vi "Expand.vi"(8 "error in (no error)":errorcluster, 10 "IB_Tree.lvclass":refnum<class "IB_Tree.lvclass">, 11 "IB_TreeProjFolder in":refnum<class "IB_Tree_Item_Proj_Folder.lvclass">) -> (0 "error out":errorcluster, 2 "first expansion?":bool, 3 "IB_TreeProjFolder out":refnum<class "IB_Tree_Item_Proj_Folder.lvclass">)   [LabVIEW 2020, in "IB_Tree_Item_Proj_Folder.lvclass"]
uses:
  <vilib>/AppBuilder/IB_Classes/Tree_Item_Proj_Folder/IB_Tree_Item_Proj_Folder.lvclass
  <vilib>/AppBuilder/IB_Classes/Tree_Item_Proj_Folder/IB_Tree_Item_Proj_Folder.lvclass/IB_Tree_Item_Proj_Folder.ctl
  <vilib>/AppBuilder/IB_Classes/Tree_Item/IB_Tree_Item.lvclass
  <vilib>/AppBuilder/IB_Classes/Tree_Item_Proj/IB_Tree_Item_Proj.lvclass
  <vilib>/AppBuilder/IB_Classes/Tree/IB_Tree.lvclass
  <vilib>/AppBuilder/IB_Classes/Tree_Item_Proj_Container/IB_Tree_Item_Proj_Container.lvclass
  e:/builds/penguin/labview/branches/2020/dev/dist/vi.lib/AppBuilder/IB_Classes/Tree_Item_Proj_Container/IB_Tree_Item_Proj_Container.lvclass
  e:/builds/penguin/labview/branches/2020/dev/dist/vi.lib/AppBuilder/IB_Classes/Tree_Item_Proj/IB_Tree_Item_Proj.lvclass
  e:/builds/penguin/labview/branches/2020/dev/dist/vi.lib/AppBuilder/IB_Classes/Tree_Item/IB_Tree_Item.lvclass
  e:/builds/penguin/labview/branches/2020/dev/dist/vi.lib/AppBuilder/IB_Classes/Tree_Item_Proj_Folder/IB_Tree_Item_Proj_Folder.lvclass
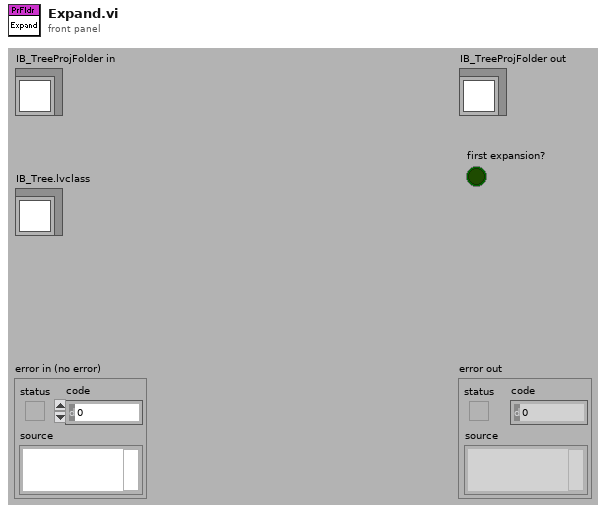
[diagram p1: front panel]
types:
  T1 = typedef "IB_Tree_Item.ctl" = cluster{"symbol index":i32, "child tag":string, "parentTag":string, "left cell name":string}
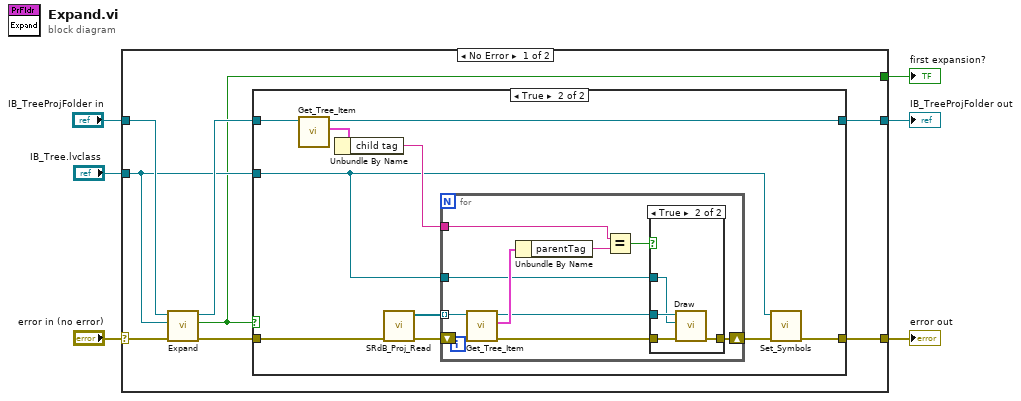
[diagram p0: block diagram]
diagram:
  n1 = case shown="No Error" "error in (no error)" {
    selector: "error in (no error)" -> [w13 w43]
    tunnel: [w7 w43] -> w6
    tunnel: [w8 _] -> w5
    tunnel: [w11 w42] -> w4
    tunnel: "IB_Tree.lvclass" -> [w9 _]
    tunnel: "IB_TreeProjFolder in" -> [w14 w42]
    frame No Error {
      n2 = call-parent "Expand.vi"("error in (no error)"=w13, "IB_Tree.lvclass"=w9, "IB_TreeRootItem in"=w14) -> ("error out"=w10:errorcluster, "first expansion?"=w8:bool, "IB_TreeRootItem out"=w12:refnum<class "IB_Tree_Item_Proj_Folder.lvclass">)  [unwired: 6 out]
      n3 = case shown="True" w8 {
        tunnel: w12 -> [w15 w25]
        tunnel: [w15 w24] -> w11
        tunnel: w10 -> [w16 w20]
        tunnel: [w16 w17] -> w7
        tunnel: w9 -> [_ w19]
        frame False {
        }
        frame True {
          n4 = call <vilib>:"Get_Tree_Item.vi"("IB_TreeItem in"=w25) -> ("data"=w23:T1, "IB_TreeItem out"=w24:refnum<class "IB_Tree_Item_Proj_Folder.lvclass">)  [unwired: 1 in, 8 out]
          n5 = Unbundle By Name(w23) -> ("child tag"=w22:string)
          n6 = call <resource>:"SRdB_Proj_Read.vi"("error in (no error)"=w20) -> ("error out"=w21:errorcluster, "Proj Items"=w26:refnum<class "IB_Tree_Item_Proj.lvclass">[])  [unwired: 9 out]
          n7 = for {
            tunnel: w26 -> [w36] mode=indexing
            tunnel: w22 -> [w34]
            shift-right: [w28] -> w18
            shift-left: w21 -> [w30]
            tunnel: w19 -> [w27]
            n8 = call <vilib>:"Get_Tree_Item.vi"("error in (no error)"=w30, "IB_TreeItem in"=w36) -> ("error out"=w29:errorcluster, "data"=w35:T1, "IB_TreeItem out"=w31:refnum<class "IB_Tree_Item_Proj.lvclass">)  [unwired: 7 out]
            n9 = Unbundle By Name(w35) -> ("parentTag"=w33:string)
            n10 = Equal?(x=w34, y=w33) -> (x = y?=w32:bool)
            n11 = case shown="True" w32 {
              tunnel: w31 -> [_ w41]
              tunnel: w29 -> [w37 w40]
              tunnel: [w37 w39] -> w28
              tunnel: w27 -> [_ w38]
              frame False {
              }
              frame True {
                n12 = call-dynamic "Draw.vi"("error in (no error)"=w40, "IB_Tree"=w38, "IB_TreeItem in"=w41) -> ("error out"=w39:errorcluster)  [unwired: 1 in, 7 out]
              }
            }
          }
          n13 = call <vilib>:"Set_Symbols.vi"("error in (no error)"=w18, "IB_Tree in"=w19) -> ("error out"=w17:errorcluster)  [unwired: 9 out]
        }
      }
    }
    frame Error {
    }
  }
  "error out" <- w6
  "IB_TreeProjFolder out" <- w4
  "first expansion?" <- w5
